vi "Check Opened.vi"(8 "error in (no error)":errorcluster, 11 "Waveform Session in":refnum<class "Waveform Session.lvclass">) -> (0 "error out":errorcluster, 3 "Waveform Session out":refnum<class "Waveform Session.lvclass">)   [LabVIEW 2020, in "NI_VS Custom Device Waveform API.lvlib" / "Waveform Session.lvclass"]
uses:
  Waveform Session.lvclass
  Waveform Session.lvclass/Waveform Session.ctl
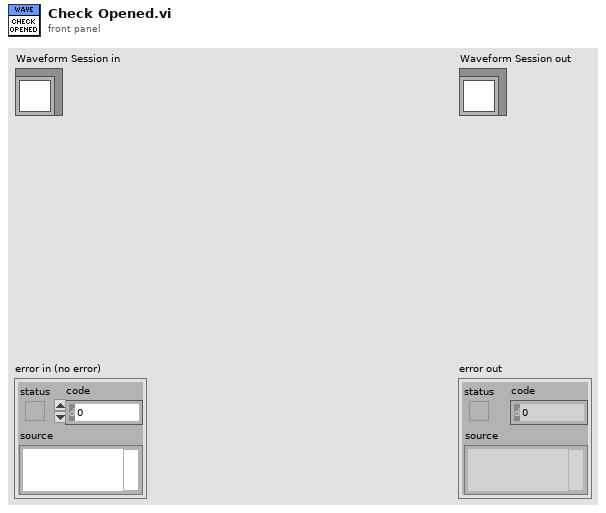
[diagram p1: front panel]
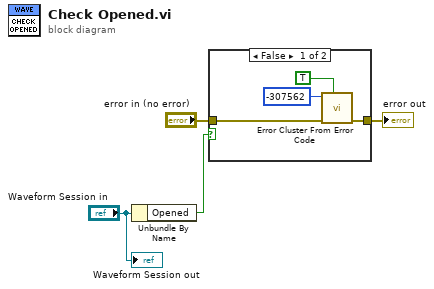
[diagram p0: block diagram]
diagram:
  n1 = Unbundle By Name("Waveform Session in") -> ("Opened"=w1:bool)
  n2 = case shown="False" w1 {
    tunnel: "error in (no error)" -> [w8 w9]
    tunnel: [w6 w9] -> w2
    frame False {
      n3 = call <vilib>:"Error Cluster From Error Code.vi"("show call chain? (False)"=TRUE, "error in (no error)"=w8, "error code (0)"=-307562) -> ("error out"=w6:errorcluster)  [unwired: 6 in]
    }
    frame True {
    }
  }
  "error out" <- w2
  "Waveform Session out" <- "Waveform Session in"
